vi "ETL Get Module.vi"(8 "error in (no error)":errorcluster, 10 "Module SN":string="https://staging-etl.app.cern.ch", 11 "Base URL":string="https://staging-etl.app.cern.ch") -> (0 "error out":errorcluster, 3 "Module Components":T1)   [LabVIEW 2024, in "ETL API.lvlib"]
uses:
  ETL API.lvlib
  ETL API Module.ctl
  ETL API Component.ctl
  <vilib>/addons/_JKI.lib/REST Client/classes/REST Client/REST Client.lvclass
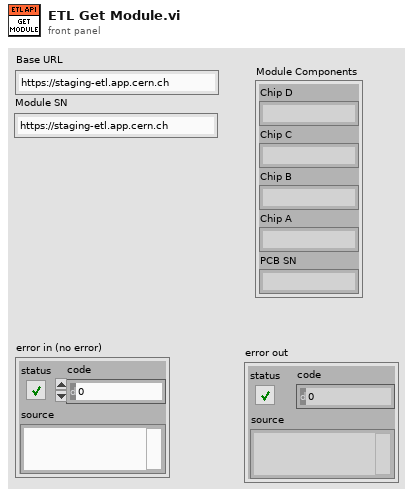
[diagram p1: front panel]
types:
  T1 = cluster{"Chip D":string, "Chip C":string, "Chip B":string, "Chip A":string, "PCB SN":string}
  T2 = typedef "ETL API.lvlib/ETL API Module.ctl" = cluster{"serial_number":string, "module_type":string, "id":dbl, "user_created":string, "assembly_location":string, "created_at":string, "current_location":string, "data":cluster{"assemblies":dbl[], "observations":dbl[], "shipments":dbl[], "tests":dbl[]}, "components":string[]}
  T3 = typedef "ETL API.lvlib/ETL API Component.ctl" = cluster{"associated_module":string, "component_pos":u32, "component_type":string, "created_at":string, "current_location":string, "id":u32, "serial_number":string, "user_created":string, "vendor":string, "data":cluster{"assemblies":dbl[], "observations":dbl[], "shipments":dbl[], "tests":dbl[]}}
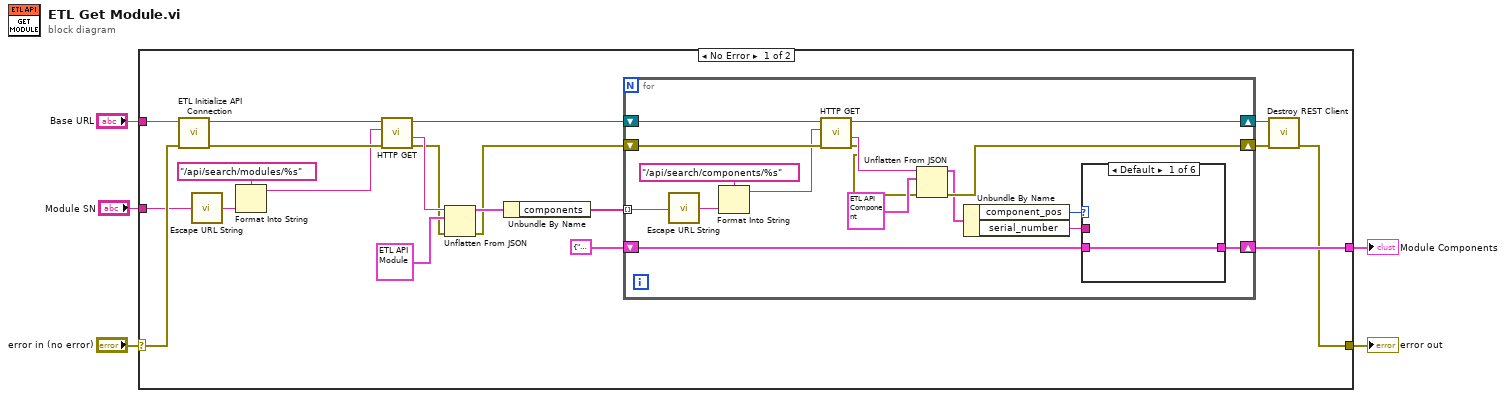
[diagram p0: block diagram]
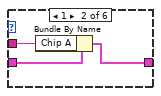
[diagram p2: hidden frame]
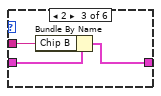
[diagram p3: hidden frame]
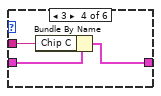
[diagram p4: hidden frame]
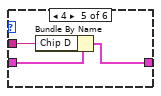
[diagram p5: hidden frame]
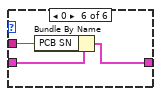
[diagram p6: hidden frame]
diagram:
  n1 = case shown="No Error" "error in (no error)" {
    selector: "error in (no error)" -> [w25 w58]
    tunnel: "Base URL" -> [w21 _]
    tunnel: [w6 w58] -> w3
    tunnel: "Module SN" -> [w11 _]
    tunnel: [w8 _] -> w1
    frame No Error {
      n2 = call "ETL Initialize API Connection.vi"("error in (no error)"=w25, "Base URL"=w21) -> ("error out"=w23:errorcluster, "REST Client out"=w24:refnum<class "REST Client.lvclass">)  [unwired: 8 in]
      n3 = call <vilib>:"Escape URL String.vi"("Unescaped URL string in"=w11) -> ("Escaped URL string out"=w10:string)
      n4 = Format Into String(format string="/api/search/modules/%s" ("string"), w10) -> (resulting string=w12:string)  [unwired: 2 in, 1 out]
      n5 = call-dynamic "HTTP GET.vi"("error in (no error)"=w23, "Path"=w12, "REST Client in"=w24) -> ("error out"=w14:errorcluster, "Response body"=w22:string, "REST Client out"=w17:refnum<class "REST Client.lvclass">)  [unwired: 3 in, 3 out]
      n6 = Unflatten From JSON(JSON string=w22, type and defaults=T2 {"serial_number"="", "module_type"="", "id"=0.0, "user_created"="", "assembly_location"="", "created_at"="", "current_location"="", "data"={"assemblies"=[], "observations"=[], "shipments"=[], "tests"=[]}, "components"=[]} ("ETL API Module"), error in (no error)=w14) -> (value=w18:T2, error out=w13:errorcluster)  [unwired: 4 in]
      n7 = Unbundle By Name(w18) -> ("components"=w16:string[])
      n8 = for {
        tunnel: w16 -> [w37] mode=indexing
        shift-right: [w39] -> w15
        shift-left: w17 -> [w41]
        shift-right: [w31] -> w7
        shift-left: w13 -> [w38]
        shift-right: [w26] -> w8
        shift-left: T1 {"Chip D"="", "Chip C"="", "Chip B"="", "Chip A"="", "PCB SN"=""} ("module_1") -> [w27]
        n9 = call <vilib>:"Escape URL String.vi"("Unescaped URL string in"=w37) -> ("Escaped URL string out"=w36:string)
        n10 = Format Into String(format string="/api/search/components/%s" ("string"), w36) -> (resulting string=w35:string)  [unwired: 2 in, 1 out]
        n11 = call-dynamic "HTTP GET.vi"("error in (no error)"=w38, "Path"=w35, "REST Client in"=w41) -> ("error out"=w32:errorcluster, "Response body"=w34:string, "REST Client out"=w39:refnum<class "REST Client.lvclass">)  [unwired: 3 in, 3 out]
        n12 = Unflatten From JSON(JSON string=w34, type and defaults=T3 {"associated_module"="", "component_pos"=0, "component_type"="", "created_at"="", "current_location"="", "id"=0, "serial_number"="", "user_created"="", "vendor"="", "data"={"assemblies"=[], "observations"=[], "shipments"=[], "tests"=[]}} ("ETL API Component"), error in (no error)=w32) -> (value=w30:T3, error out=w31:errorcluster)  [unwired: 4 in]
        n13 = Unbundle By Name(w30) -> ("component_pos"=w29:u32, "serial_number"=w28:string)
        n14 = case shown="Default" w29 {
          tunnel: w28 -> [_ w43 w46 w49 w52 w55]
          tunnel: w27 -> [w42 w45 w48 w51 w54 w57]
          tunnel: [w42 w44 w47 w50 w53 w56] -> w26
          frame Default {
          }
          frame 1 {
            n15 = Bundle By Name(cluster=w45, "Chip A"=w43) -> (w44:T1)
          }
          frame 2 {
            n16 = Bundle By Name(cluster=w48, "Chip B"=w46) -> (w47:T1)
          }
          frame 3 {
            n17 = Bundle By Name(cluster=w51, "Chip C"=w49) -> (w50:T1)
          }
          frame 4 {
            n18 = Bundle By Name(cluster=w54, "Chip D"=w52) -> (w53:T1)
          }
          frame 0 {
            n19 = Bundle By Name(cluster=w57, "PCB SN"=w55) -> (w56:T1)
          }
        }
      }
      n20 = call-dynamic "Destroy REST Client.vi"("error in (no error)"=w7, "REST Client in"=w15) -> ("error out"=w6:errorcluster)  [unwired: 9 in]
    }
    frame Error {
    }
  }
  "error out" <- w3
  "Module Components" <- w1
